vi "Configure Measurement (Baseband Noise).vi"(0 "VISA resource name":refnum<visa-resource-name>, 1 "Spurious Mode (0: Normalized)":u16(ring) items=["Normalized (dBc/Hz)", "Power (dBc)", "Omit"], 5 "Intermediate Frequency Gain (20 dB)":i32=20 format="%^#_9g", 7 "Correlation (1)":i32=1 format="%^#_9g", 9 "Cutoff Frequency (0: Low)":u16(ring) items=["Low", "High"], 11 "error in (no error)":errorcluster, 12 "Minimum Spur Level (-500 dBc)":dbl=-500.0 format="%^#_9g") -> (4 "VISA resource name out":refnum<visa-resource-name>, 15 "error out":errorcluster)   [LabVIEW 2011, in "Agilent E5052X.lvlib"]
doc: "Configures the instrument to take Baseband Noise measurements.\n\n<b>Note: </b>\n\n1) Baseband Measurement is not available for the E5052A signal source analyzer.\n\n2) \"Configure Measurement Characteristics(Baseband Noise)\" VI must be called before calling this VI."
uses:
  Agilent E5052X.lvlib
panel:
  # "Spurious Settings"
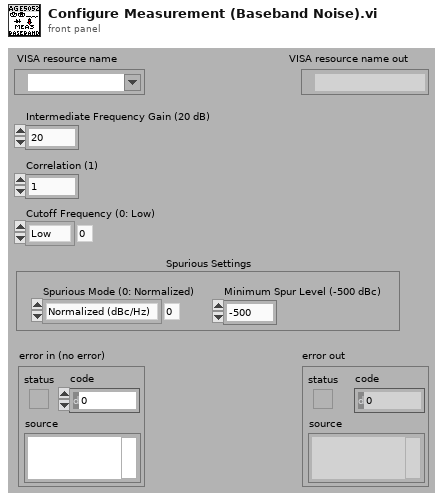
[diagram p1: front panel]
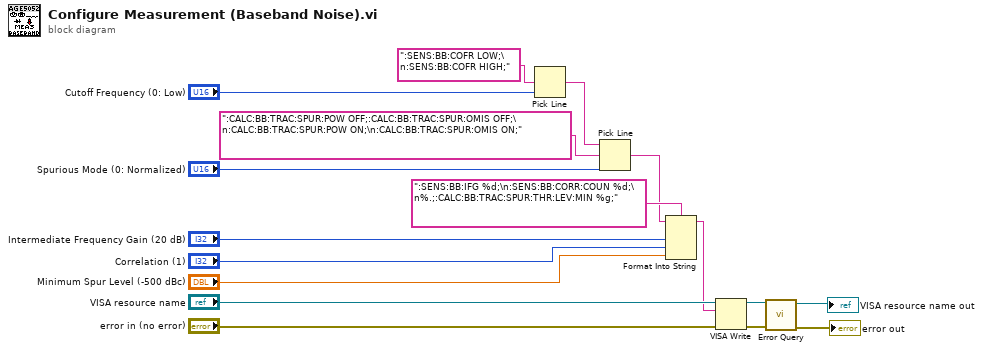
[diagram p0: block diagram]
diagram:
  n1 = Pick Line(multi-line string=":SENS:BB:COFR LOW;\n:SENS:BB:COFR HIGH;", line index="Cutoff Frequency (0: Low)") -> (output string=w3:string)  [unwired: 1 in]
  n2 = Pick Line(string ("")=w3, multi-line string=":CALC:BB:TRAC:SPUR:POW OFF;:CALC:BB:TRAC:SPUR:OMIS OFF;\n:CALC:BB:TRAC:SPUR:POW ON;\n:CALC:BB:TRAC:SPUR:OMIS ON;", line index="Spurious Mode (0: Normalized)") -> (output string=w2:string)
  n3 = Format Into String(format string=":SENS:BB:IFG %d;\n:SENS:BB:CORR:COUN %d;\n%.;:CALC:BB:TRAC:SPUR:THR:LEV:MIN %g;", initial string=w2, "Intermediate Frequency Gain (20 dB)", "Correlation (1)", "Minimum Spur Level (-500 dBc)") -> (resulting string=w1:string)  [unwired: 1 in, 1 out]
  n4 = VISA Write(VISA resource name="VISA resource name", write buffer=w1, error in (no error)="error in (no error)") -> (VISA resource name out=w11:refnum<visa-resource-name>, error out=w10:errorcluster)  [unwired: 1 out]
  n5 = call "Error Query.vi"("error in (no error)"=w10, "VISA resource name"=w11) -> ("error out"=→"error out":errorcluster, "VISA resource name out"=→"VISA resource name out":refnum<visa-resource-name>)  [unwired: 6 in, 2 out]
